vi "Read_Value_From_Excel.vi"(2 "error in (no error)":errorcluster, 3 "Selected Cell":string="A1", 4 "Work Sheet":i32=1, 5 "Excel File Path":path) -> (0 "error out":errorcluster, 1 "Data from Cell":dbl format="%.2f")   [LabVIEW 2014]
doc: "This example program demonstrates how to read a value from a particular cell in an Excel spreadsheet. Specify the path to an excel file, the worksheet number, and the cell to read and run the VI. The data in the specified file will appear on the front panel."
panel:
  # "Select Help»Show Context Help and move the cursor over the VI icon to display help for this VI"
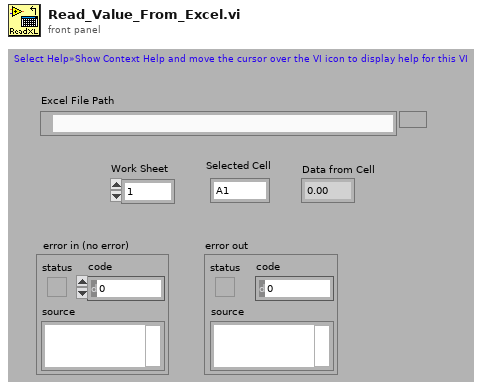
[diagram p1: front panel]
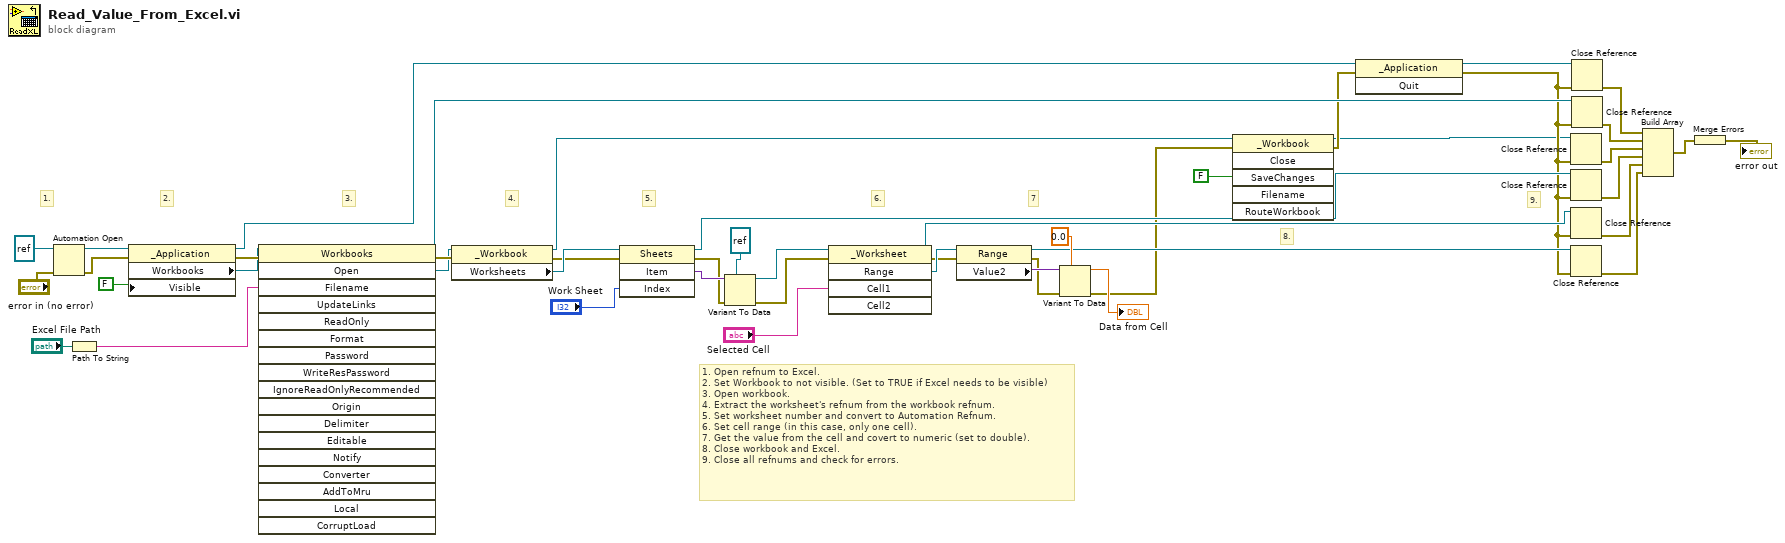
[diagram p0: block diagram]
diagram:
  # "1. Open refnum to Excel.\n2. Set Workbook to not visible. (Set to TRUE if Excel needs to be visible)\n3. Open workbook.\n4. Extract the worksheet's refnum from the workbook refnum.\n5. Set worksheet number and convert to Automation Refnum.\n6. Set cell range (in this case, only one cell).\n7. Get the value from the cell and covert to numeric (set to double).\n8. Close workbook and Excel.\n9. Close all refnums and check for errors."
  # "9."
  # "8."
  # "7"
  # "6."
  # "5."
  # "4."
  # "3."
  # "2."
  # "1."
  n1 = Automation Open(error in (no error)="error in (no error)", Automation Refnum=refnum<k7> refnum ("Excel._Application")) -> (Automation Refnum=w44:refnum<k7>, error out=w43:errorcluster)  [unwired: 2 in]
  n2 = Path To String(path="Excel File Path") -> (string=w38:string)
  n3 = property class="_Application"(reference=w44, error in=w43, "Visible"=FALSE) -> (reference out=w4:refnum<k7>, error out=w41:errorcluster, "Workbooks"=w40:refnum<k7>)
  n4 = invoke class="Workbooks" method="Open"(reference=w40, error in=w41, "Filename"=w38) -> (reference out=w20:refnum<k7>, error out=w37:errorcluster, "Open"=w36:refnum<k7>)  [unwired: 15 in, 15 out]
  n5 = property class="_Workbook"(reference=w36, error in=w37) -> (reference out=w8:refnum<k7>, error out=w33:errorcluster, "Worksheets"=w34:refnum<k7>)
  n6 = invoke class="Sheets" method="Item"(reference=w34, error in=w33, "Index"="Work Sheet") -> (reference out=w19:refnum<k7>, error out=w30:errorcluster, "Item"=w31:variant)  [unwired: 1 in, 1 out]
  n7 = Variant To Data(error in=w30, type=refnum<k7> refnum ("Excel._Worksheet"), Variant=w31) -> (data=w29:refnum<k7>, error out=w28:errorcluster)
  n8 = invoke class="_Worksheet" method="Range"(reference=w29, error in=w28, "Cell1"="Selected Cell") -> (reference out=w18:refnum<k7>, error out=w25:errorcluster, "Range"=w26:refnum<k7>)  [unwired: 2 in, 2 out]
  n9 = property class="Range"(reference=w26, error in=w25) -> (reference out=w17:refnum<k7>, error out=w23:errorcluster, "Value2"=w24:variant)
  n10 = Variant To Data(error in=w23, type=0.0, Variant=w24) -> (data=→"Data from Cell":dbl, error out=w6:errorcluster)
  n11 = invoke class="_Workbook" method="Close"(reference=w8, error in=w6, "SaveChanges"=FALSE) -> (reference out=w1:refnum<k7>, error out=w3:errorcluster)  [unwired: 3 in, 4 out]
  n12 = invoke class="_Application" method="Quit"(reference=w4, error in=w3) -> (reference out=w5:refnum<k7>, error out=w2:errorcluster)  [unwired: 1 in, 1 out]
  n13 = Close Reference(reference=w1, error in (no error)=w2) -> (error out=w14:errorcluster)
  n14 = Close Reference(reference=w19, error in (no error)=w2) -> (error out=w13:errorcluster)
  n15 = Close Reference(reference=w18, error in (no error)=w2) -> (error out=w12:errorcluster)
  n16 = Close Reference(reference=w17, error in (no error)=w2) -> (error out=w11:errorcluster)
  n17 = Close Reference(reference=w5, error in (no error)=w2) -> (error out=w16:errorcluster)
  n18 = Close Reference(reference=w20, error in (no error)=w2) -> (error out=w15:errorcluster)
  n19 = Build Array(w16, w15, w14, w13, w12, w11) -> (w10:errorcluster[])
  n20 = Merge Errors(w10) -> (→"error out":errorcluster)
